vi "PolyLaguerreAsso.vi"(1 "alpha":dbl, 2 "n":i32) -> (0 "Lna":dbl[](array[numeric]))   [LabVIEW 2014, in "NI_AALPro.lvlib"]
uses:
  NI_AALPro.lvlib
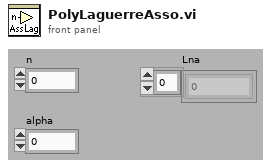
[diagram p1: front panel]
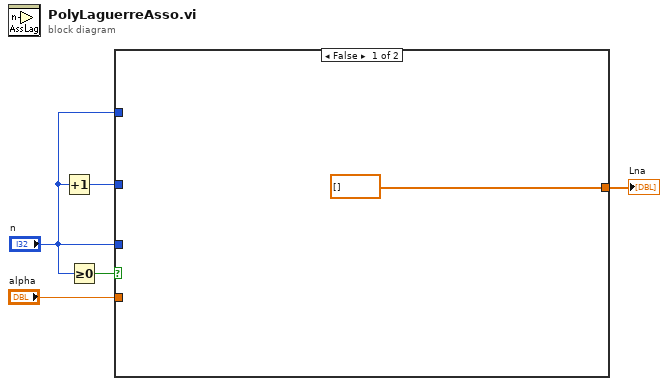
[diagram p0: block diagram]
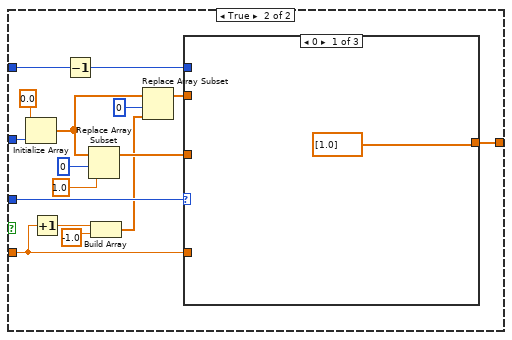
[diagram p2: hidden frame]
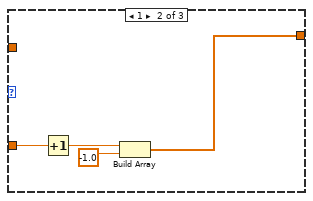
[diagram p3: hidden frame]
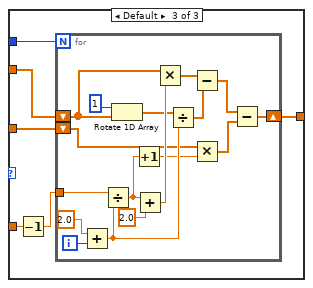
[diagram p4: hidden frame]
diagram:
  n1 = Increment(x="n") -> (x+1=w4:i32)
  n2 = Greater Or Equal To 0?(x="n") -> (x >= 0?=w5:bool)
  n3 = case shown="False" w5 {
    tunnel: "n" -> [_ w22]
    tunnel: w4 -> [_ w16]
    tunnel: "n" -> [_ w14]
    tunnel: [dbl[] [] ("Tn(x)") w15] -> w2
    tunnel: "alpha" -> [_ w10]
    frame False {
    }
    frame True {
      n4 = Initialize Array(0.0 ("element"), w16) -> (w12:dbl[])
      n5 = Increment(x=w10) -> (x+1=w9:dbl)
      n6 = Decrement(x=w14) -> (x-1=w13:i32)
      n7 = Replace Array Subset(array=w12, new element=1.0 ("new element/subarray"), index=0) -> (w11:dbl[])
      n8 = Build Array(w9, -1.0 ("element")) -> (w7:dbl[])
      n9 = Replace Array Subset(array=w12, new element=w7, index=0) -> (w17:dbl[])
      n10 = case shown="0" w22 {
        tunnel: w17 -> [_ _ w33]
        tunnel: w11 -> [_ _ w32]
        tunnel: w13 -> [_ _ w31]
        tunnel: [dbl[] [1.0] ("Tn(x)") w24 w30] -> w15
        tunnel: w10 -> [_ w27 w29]
        frame 0 {
        }
        frame 1 {
          n11 = Increment(x=w27) -> (x+1=w26:dbl)
          n12 = Build Array(w26, -1.0 ("element")) -> (w24:dbl[])
        }
        frame Default {
          n13 = Decrement(x=w29) -> (x-1=w28:dbl)
          n14 = for {
            N: w31 -> [_]
            shift-right: [w36] -> w30
            shift-left: w33 -> [w45]
            shift-left: w32 -> [w37]
            tunnel: w28 -> [w47]
            i -> [w49]
            n15 = Add(x=2.0, y=w49) -> (x+y=w41:dbl)
            n16 = Divide(x=w47, y=w41) -> (x/y=w39:dbl)
            n17 = Rotate 1D Array(1:w45, 2:1 ("n")) -> (0:w42:dbl[])
            n18 = Increment(x=w39) -> (x+1=w38:dbl)
            n19 = Add(x=w39, y=2.0) -> (x+y=w44:dbl)
            n20 = Multiply(x=w45, y=w44) -> (x*y=w43:dbl[])
            n21 = Divide(x=w42, y=w41) -> (x/y=w40:dbl[])
            n22 = Subtract(x=w43, y=w40) -> (x-y=w35:dbl[])
            n23 = Multiply(x=w37, y=w38) -> (x*y=w34:dbl[])
            n24 = Subtract(x=w35, y=w34) -> (x-y=w36:dbl[])
          }
        }
      }
    }
  }
  "Lna" <- w2
